vi "matrix multiplication.vi"() -> ()   [LabVIEW 2019]
uses:
  <vilib>/Analysis/Matrix/Datatypes/RealMatrix.ctl
  <vilib>/Analysis/Matrix/Numeric/Multiply/Multiply - RM,RM.vi
  <vilib>/Analysis/Matrix/NI_Matrix.lvlib
panel:
  in  "?":bool
  out "Matrix 3":dbl[][](array[numeric])
  in  "Matrix 2":dbl[][](array[numeric])
  in  "Matrix 1":dbl[][](array[numeric])
  # "matrix multiplication"
  # "x"
  # "="
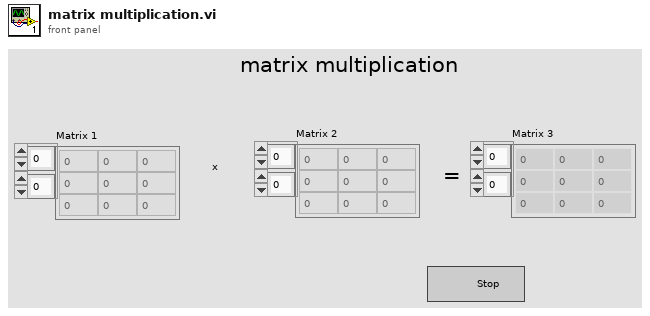
[diagram p1: front panel]
types:
  T1 = typedef "NI_Matrix.lvlib/RealMatrix.ctl" = dbl[][]
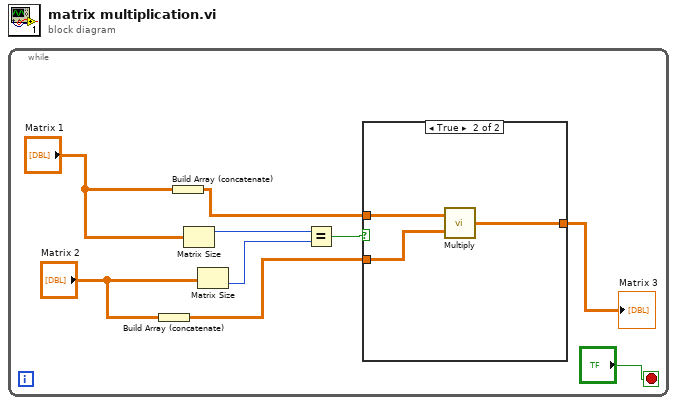
[diagram p0: block diagram]
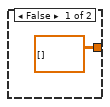
[diagram p2: hidden frame]
diagram:
  n1 = while {
    stop <- "?" stop-if-true
    n2 = Build Array (concatenate)("Matrix 2") -> (w3:T1)
    n3 = Build Array (concatenate)("Matrix 1") -> (w4:T1)
    n4 = Matrix Size(0:"Matrix 1") -> (1:w7:i32)  [unwired: 1 out]
    n5 = Matrix Size(0:"Matrix 2") -> (2:w6:i32)  [unwired: 1 out]
    n6 = Equal?(x=w7, y=w6) -> (x = y?=w5:bool)
    n7 = case shown="True" w5 {
      tunnel: w4 -> [_ w13]
      tunnel: w3 -> [_ w12]
      tunnel: [T1 [] ("A * B") w11] -> w2
      frame False {
      }
      frame True {
        n8 = call-poly <vilib>:"Multiply.vi"("Real Matrix B"=w12, "Real Matrix A"=w13) -> ("A * B"=w11:T1)
      }
    }
    "Matrix 3" <- w2
  }
